vi "Configure Active Trace.vi"(5 "Format":T1, 7 "S parameter":T2(ring), 8 "error in (no error)":errorcluster, 10 "Active Trace":u8=1, 11 "VNA-Keysight PNA in":refnum<class "VNA-Keysight PNA.lvclass">) -> (0 "error out":errorcluster, 3 "VNA-Keysight PNA out":refnum<class "VNA-Keysight PNA.lvclass">)   [LabVIEW 2020, in "VNA-Keysight PNA.lvclass"]
doc: "Configures the active trace.\nIt creates the trace and sets the S paramert and mode."
uses:
  VNA-Keysight PNA.lvclass
  C:/Sandbox/Git_Sandbox/WiSpry Test Framework source code (LV20)/WiSpry Test Framework/Instruments/Vector Network Analyzer/Vector Network Analyzer.lvclass
  C:/Sandbox/Git_Sandbox/WiSpry Test Framework source code (LV20)/WiSpry Test Framework/Instruments/Instrument.lvclass
  Controls/S parm format enum.ctl
  Vector Network Analyzer.lvclass/Vector Network Analyzer.ctl
  Instrument.lvclass/Instrument.ctl
  Vector Network Analyzer.lvclass
  Instrument.lvclass
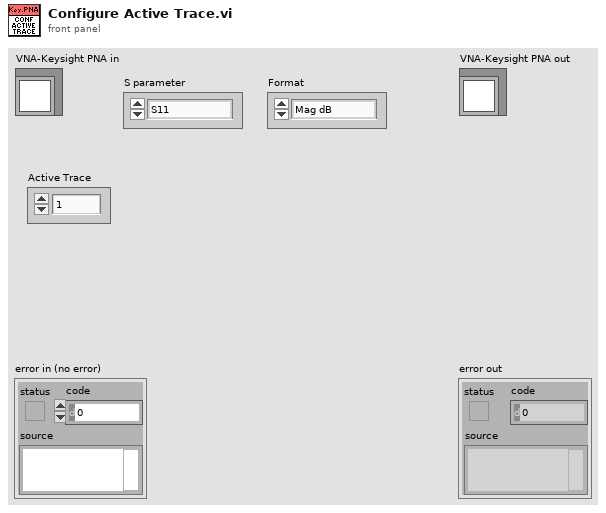
[diagram p1: front panel]
types:
  T1 = typedef "Vector Network Analyzer.lvclass/S parm format enum.ctl" = enum16{"Mag dB", "Mag", "Phase", "Smith", "Real", "Imag", "Group Delay", "SWR"}
  T2 = enum16{"S11", "S21", "S31", "S41", "S22", "S12", "S32", "S42", "S33", "S13", "S23", "S43", "S44", "S14", "S24", "S34"}
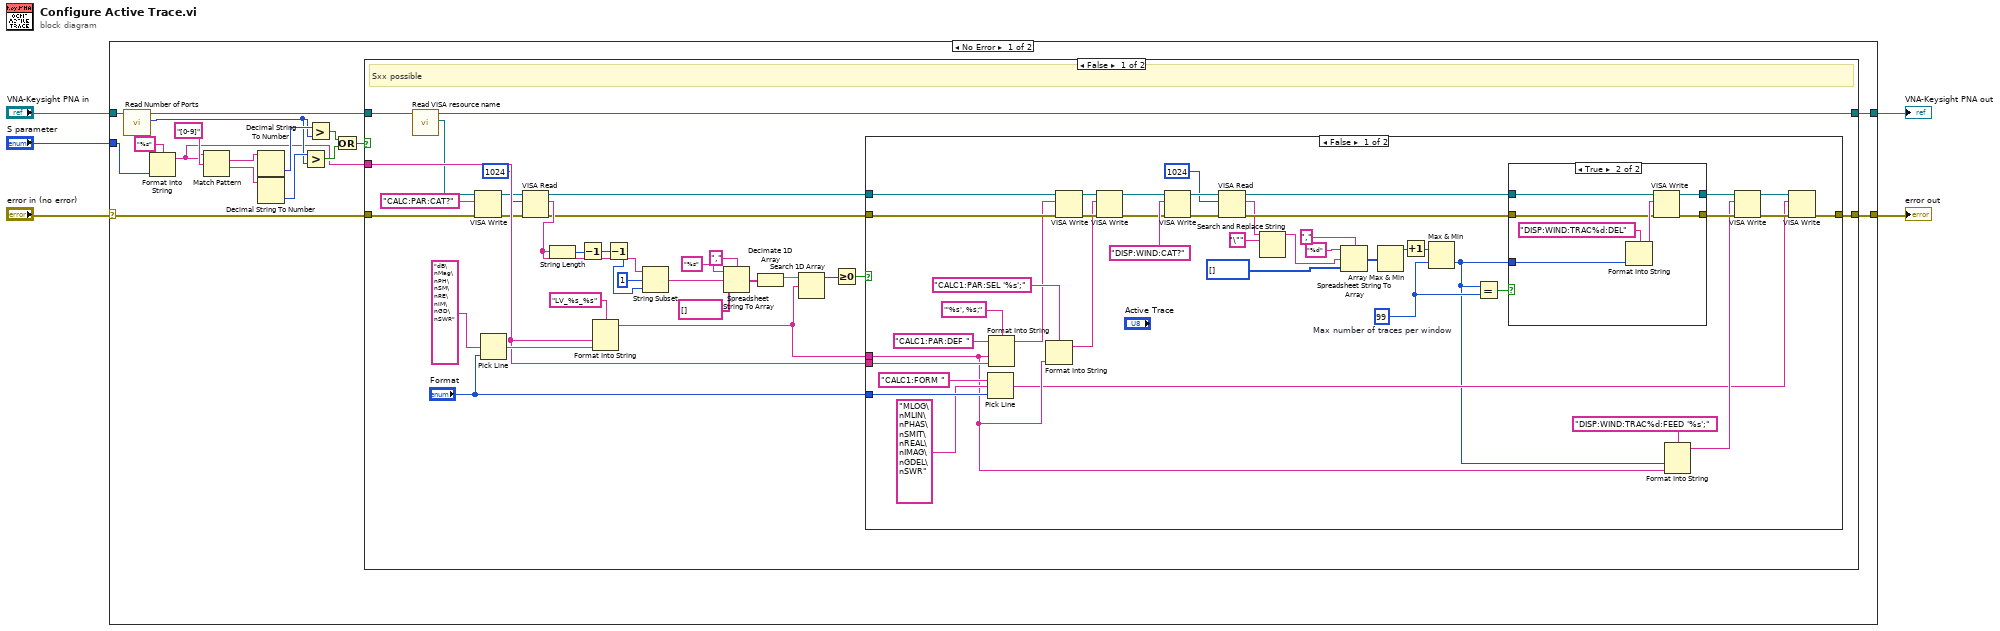
[diagram p0: block diagram]
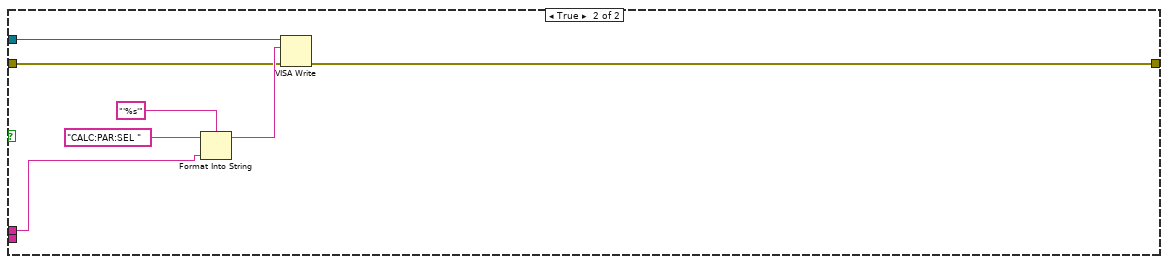
[diagram p3: hidden frame]
diagram:
  n1 = case shown="No Error" "error in (no error)" {
    selector: "error in (no error)" -> [w9 w114]
    tunnel: "VNA-Keysight PNA in" -> [w22 w113]
    tunnel: "S parameter" -> [w20 _]
    tunnel: [w7 w114] -> w5
    tunnel: [w6 w113] -> w4
    frame No Error {
      n2 = call "Read Number of Ports.vi"("Vector Network Analyzer in"=w22) -> ("Number of Ports"=w14:i32, "Vector Network Analyzer out"=w10:refnum<class "VNA-Keysight PNA.lvclass">)  [unwired: 9 in]
      n3 = Format Into String(format string="%s", w20) -> (resulting string=w8:string)  [unwired: 2 in, 1 out]
      n4 = Match Pattern(string=w8, regular expression="[0-9]") -> (match substring=w18:string, after substring=w17:string)  [unwired: 1 in, 2 out]
      n5 = Decimal String To Number(string=w18) -> (number=w16:i32)  [unwired: 2 in, 1 out]
      n6 = Decimal String To Number(string=w17) -> (number=w15:i32)  [unwired: 2 in, 1 out]
      n7 = Greater?(x=w15, y=w14) -> (0:w12:bool)
      n8 = Greater?(x=w16, y=w14) -> (0:w13:bool)
      n9 = Or(x=w13, y=w12) -> (x .or. y?=w11:bool)
      n10 = case shown="False" w11 {
        tunnel: w10 -> [w51 w112]
        tunnel: w9 -> [w44 w111]
        tunnel: w8 -> [w46 _]
        tunnel: [w47 w111] -> w7
        tunnel: [w50 w112] -> w6
        frame False {
          # "Sxx possible"
          n11 = call "Read VISA resource name.vi"("Instrument in"=w51) -> ("VISA resource name"=w45:refnum<visa-resource-name>, "Instrument out"=w50:refnum<class "VNA-Keysight PNA.lvclass">)  [unwired: 9 in]
          n12 = VISA Write(VISA resource name=w45, write buffer="CALC:PAR:CAT?", error in (no error)=w44) -> (VISA resource name out=w41:refnum<visa-resource-name>, error out=w42:errorcluster)  [unwired: 1 out]
          n13 = Pick Line(multi-line string="dB\nMag\nPH\nSM\nRE\nIM\nGD\nSWR", line index="Format") -> (output string=w48:string)  [unwired: 1 in]
          n14 = VISA Read(VISA resource name=w41, byte count=u32 1024, error in (no error)=w42) -> (VISA resource name out=w28:refnum<visa-resource-name>, read buffer=w36:string, error out=w30:errorcluster)  [unwired: 1 out]
          n15 = String Length(string=w36) -> (length=w37:i32)
          n16 = Decrement(x=w37) -> (x-1=w24:i32)
          n17 = Format Into String(format string="LV_%s_%s" ("initial string"), w46, w48) -> (resulting string=w27:string)  [unwired: 2 in, 1 out]
          n18 = Decrement(x=w24) -> (x-1=w23:i32)
          n19 = String Subset(string=w36, offset (0)=1, length (rest)=w23) -> (substring=w34:string)
          n20 = Spreadsheet String To Array(delimiter (Tab)=",", format string="%s", spreadsheet string=w34, array type (2D Dbl)=string[] []) -> (array=w31:string[])
          n21 = Decimate 1D Array(w31) -> (w26:string[])  [unwired: 1 out]
          n22 = Search 1D Array(1D array=w26, element=w27) -> (index of element=w32:i32)  [unwired: 1 in]
          n23 = Greater Or Equal To 0?(x=w32) -> (x >= 0?=w29:bool)
          n24 = case shown="False" w29 {
            tunnel: [w62 w104] -> w47
            tunnel: w46 -> [w94 _]
            tunnel: "Format" -> [w93 _]
            tunnel: w27 -> [w86 w107]
            tunnel: w30 -> [w85 w106]
            tunnel: w28 -> [w84 w105]
            frame False {
              w55 = 99  # Max number of traces per window
              n25 = Pick Line(string ("")="CALC1:FORM ", multi-line string="MLOG\nMLIN\nPHAS\nSMIT\nREAL\nIMAG\nGDEL\nSWR", line index=w93) -> (output string=w59:string)
              n26 = Format Into String(format string="'%s', %s;", initial string="CALC1:PAR:DEF ", w86, w94) -> (resulting string=w83:string)  [unwired: 1 in, 1 out]
              n27 = Format Into String(format string="CALC1:PAR:SEL '%s';", w86) -> (resulting string=w80:string)  [unwired: 2 in, 1 out]
              n28 = VISA Write(VISA resource name=w84, write buffer=w83, error in (no error)=w85) -> (VISA resource name out=w81:refnum<visa-resource-name>, error out=w82:errorcluster)  [unwired: 1 out]
              n29 = VISA Write(VISA resource name=w81, write buffer=w80, error in (no error)=w82) -> (VISA resource name out=w64:refnum<visa-resource-name>, error out=w65:errorcluster)  [unwired: 1 out]
              n30 = VISA Write(VISA resource name=w64, write buffer="DISP:WIND:CAT?", error in (no error)=w65) -> (VISA resource name out=w77:refnum<visa-resource-name>, error out=w78:errorcluster)  [unwired: 1 out]
              n31 = VISA Read(VISA resource name=w77, byte count=u32 1024, error in (no error)=w78) -> (VISA resource name out=w73:refnum<visa-resource-name>, read buffer=w68:string, error out=w72:errorcluster)  [unwired: 1 out]
              n32 = Search and Replace String(input string=w68, search string="\"") -> (result string=w67:string)  [unwired: 6 in, 3 out]
              n33 = Spreadsheet String To Array(delimiter (Tab)=",", format string="%d", spreadsheet string=w67, array type (2D Dbl)=i32[] []) -> (array=w58:i32[])
              n34 = Array Max & Min(array=w58) -> (max value=w57:i32)  [unwired: 3 out]
              n35 = Increment(x=w57) -> (x+1=w56:i32)
              n36 = Max & Min(x=w56, y=w55) -> (min(x,y)=w53:i32)  [unwired: 1 out]
              n37 = Equal?(x=w53, y=w55) -> (x = y?=w54:bool)
              n38 = case shown="True" w54 {
                tunnel: w73 -> [w95 w98]
                tunnel: w72 -> [w96 w99]
                tunnel: [w96 w101] -> w71
                tunnel: [w95 w97] -> w70
                tunnel: w53 -> [_ w102]
                frame False {
                }
                frame True {
                  n39 = Format Into String(format string="DISP:WIND:TRAC%d:DEL", w102) -> (resulting string=w100:string)  [unwired: 2 in, 1 out]
                  n40 = VISA Write(VISA resource name=w98, write buffer=w100, error in (no error)=w99) -> (VISA resource name out=w97:refnum<visa-resource-name>, error out=w101:errorcluster)  [unwired: 1 out]
                }
              }
              n41 = Format Into String(format string="DISP:WIND:TRAC%d:FEED '%s';" ("write buffer"), w53, w86) -> (resulting string=w63:string)  [unwired: 2 in, 1 out]
              n42 = VISA Write(VISA resource name=w70, write buffer=w63, error in (no error)=w71) -> (VISA resource name out=w60:refnum<visa-resource-name>, error out=w61:errorcluster)  [unwired: 1 out]
              n43 = VISA Write(VISA resource name=w60, write buffer=w59, error in (no error)=w61) -> (error out=w62:errorcluster)  [unwired: 2 out]
            }
            frame True {
              n44 = Format Into String(format string="'%s'", initial string="CALC:PAR:SEL ", w107) -> (resulting string=w108:string)  [unwired: 1 in, 1 out]
              n45 = VISA Write(VISA resource name=w105, write buffer=w108, error in (no error)=w106) -> (error out=w104:errorcluster)  [unwired: 2 out]
            }
          }
        }
        frame True {
          # "Add error handler"
          # "Sxx higher than ports"
        }
      }
    }
    frame Error {
    }
  }
  "error out" <- w5
  "VNA-Keysight PNA out" <- w4
